vi "LV FPGA Serial Write.vi"(0 "Transmit":refnum<k21>="Port8/DIO0", 1 "Write FIFO":refnum<k21>="Write FIFO", 7 "baud rate (9600)":u32=9600, 9 "data bits (8)":i32=8 min=5 max=8 step=1, 11 "parity (0:none)":enum16{"None", "Odd", "Even", "Mark", "Space"}(ring), 12 "stop bits (10: 1 bit)":u16(ring)=10 items=["1.0"=10, "1.5"=15, "2.0"=20], 13 "Invert Polarity?":bool) -> ()   [LabVIEW 2009]
uses:
  <vilib>/eio/EIOMethodNode/EIOMethodNode.xnode
  <vilib>/rvi/eio/nirviEIOMethodImplementation/nirviEIOMethodImplementation.xnode
  <vilib>/rvi/eio/common/nirviEmuTemplateMethod_noerrors.vi
  <vilib>/rvi/eio/common/nirviEmuClasses.ctl
  <vilib>/rvi/DataTransferAndStorage/Container/XNode/niFpgaContainer.xnode
  <vilib>/rvi/DataTransferAndStorage/Container/Common/niFpgaContainerMethod.ctl
  <vilib>/rvi/DataTransferAndStorage/Container/Common/niFpgaContainerExecOnDevCompGetState.vi
  <vilib>/rvi/DataTransferAndStorage/Container/Common/niFpgaContainerMetaDataKey.ctl
  <vilib>/rvi/FIFO/Fifo_Resource/nirvififoUniquifyingName.vi
  <vilib>/rvi/interface/RandomDataEmulation/niFpgaRandomDataHandleErrors.vi
  <vilib>/rvi/interface/RandomDataEmulation/nirviRandomDataFPGAFIFO.vi
  <vilib>/rvi/DataTransferAndStorage/Container/Common/niFpgaTransferTypeControl.ctl
  <vilib>/rvi/DataTransferAndStorage/FIFO/niFpgaPeerToPeerStreamState.ctl
  <vilib>/rvi/eio/common/nirviEmuReportErrorAndStop.vi
  <vilib>/eio/EIONode/EIONode.xnode
  <vilib>/rvi/eio/nirviEIOImplementation/nirviEIOImplementation.xnode
panel:
  out "Read: Transmission Error":bool
  in  "stop":bool
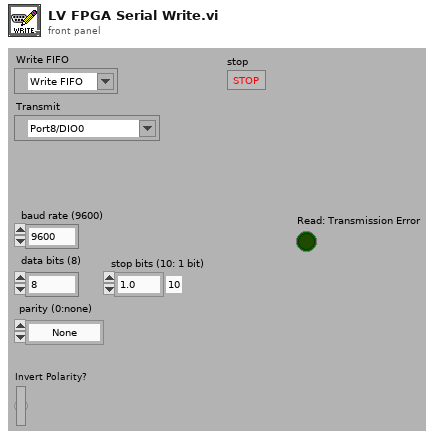
[diagram p1: front panel]
types:
  T1 = typedef "nirviEmuClasses.ctl" = enum16{"IO Read", "IO Write", "Method", "Property Read", "Property Write"}
  T2 = typedef "niFpgaContainerMethod.ctl" = enum16{"Write", "Read", "Clear", "Get Number of Elements to Write", "Get Number of Elements to Read", "Enable", "Disable", "Flush and Disable", "Get Stream State"}
  T3 = typedef "niFpgaTransferTypeControl.ctl" = enum16{"Target-Scoped", "Host to Target - DMA", "Target to Host - DMA", "Peer to Peer Reader", "Peer to Peer Writer", "Bidirectional"}
  T4 = typedef "niFpgaPeerToPeerStreamState.ctl" = enum16{"Unlinked", "Disabled", "Enabled", "Flushing"}
  T5 = typedef "niFpgaContainerMetaDataKey.ctl" = enum16{"FPGA FIFO", "FPGA Memory", "FPGA Register"}
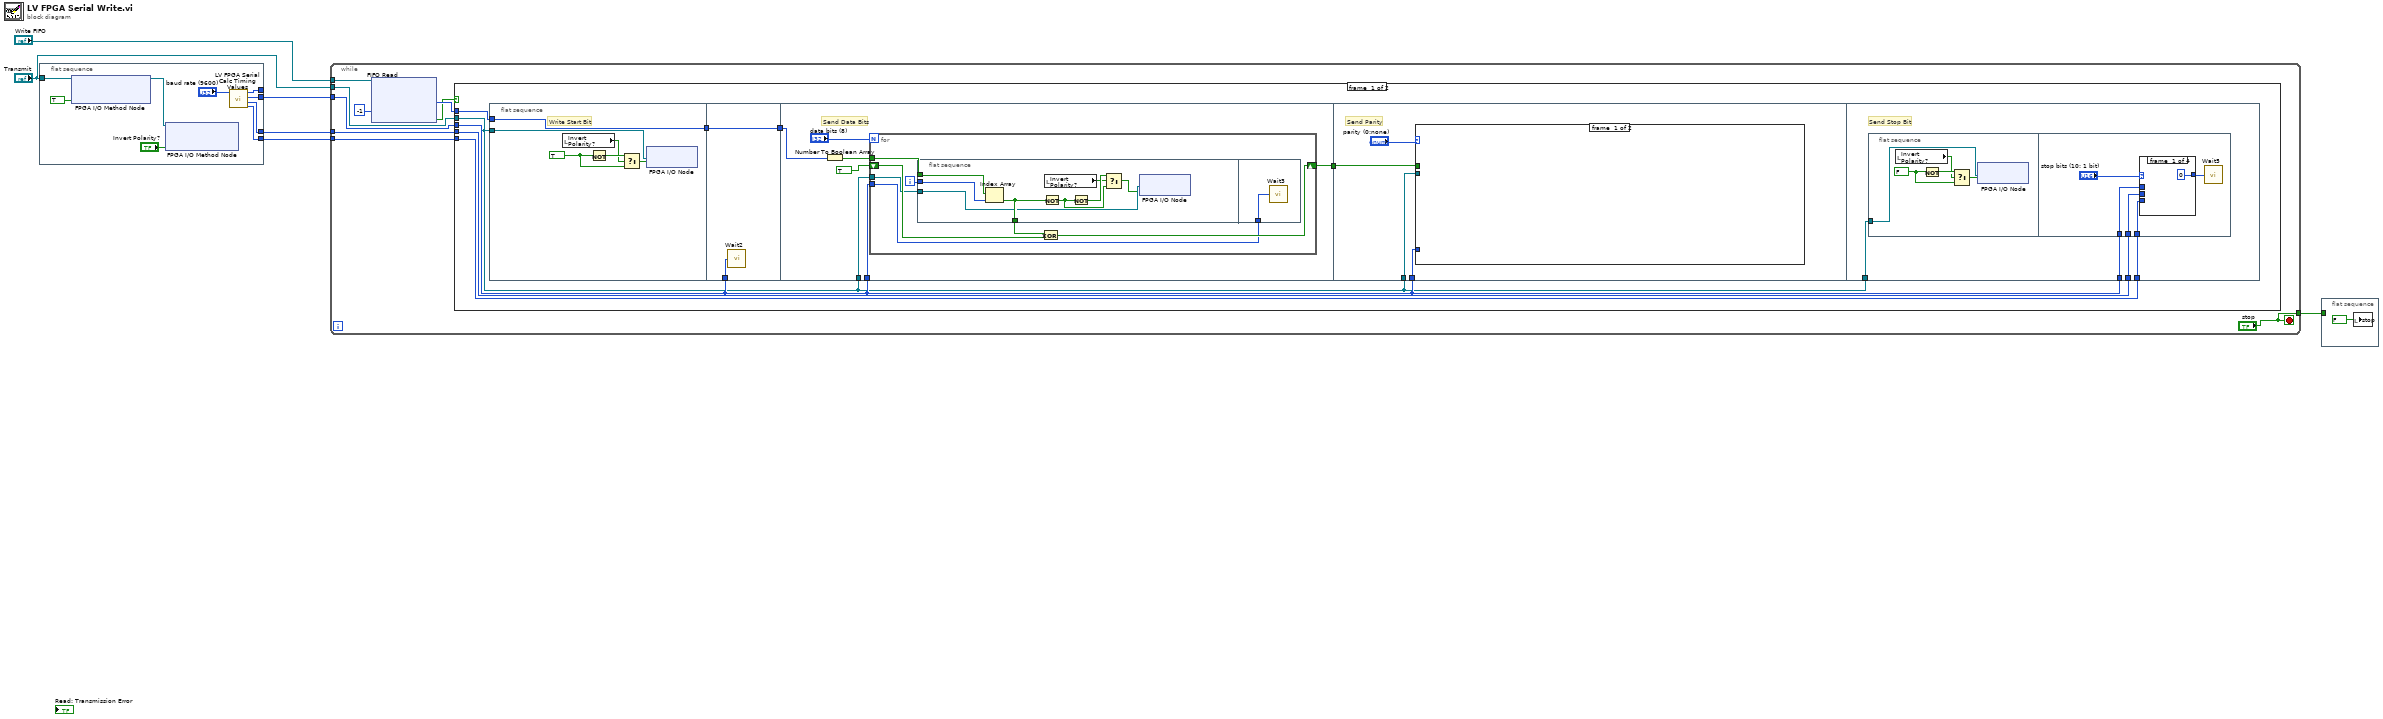
[diagram p0: block diagram]
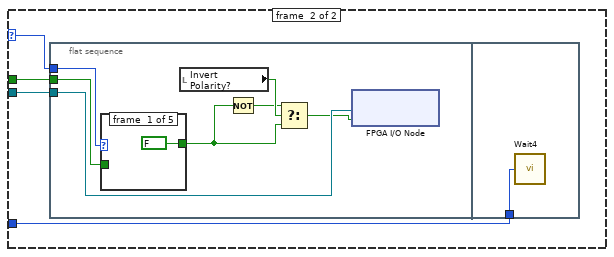
[diagram p2: hidden frame]
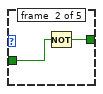
[diagram p3: hidden frame]
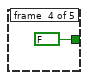
[diagram p5: hidden frame]
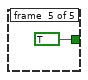
[diagram p6: hidden frame]
diagram:
  n1 = flat-sequence {
    tunnel: [w11] -> w6
    tunnel: [w14] -> _
    tunnel: [w13] -> w5
    tunnel: [w12] -> w4
    tunnel: "Transmit" -> [w9]
    frame #0 {
      n2 = xnode "FPGA I/O Method Node"("FPGA I/O In"=w9, "Enable"=TRUE ("Digital Enable")) -> ("FPGA I/O Out"=w8:refnum<k21>)
      n3 = xnode "FPGA I/O Method Node"("FPGA I/O In"=w8, "Data"="Invert Polarity?") -> ()  [unwired: 1 out]
      n4 = call "LV FPGA Serial Calc Timing Values.vi"("baud rate (1000000)"="baud rate (9600)") -> ("Two Bit"=w12:u32, "One and Half Bit"=w13:u32, "One Bit"=w11:u32, "Half Bit"=w14:u32)  [unwired: 1 in, 2 out]
    }
  }
  n5 = while {
    tunnel: w4 -> [w46]
    tunnel: w5 -> [w45]
    tunnel: w6 -> [w44]
    tunnel: "Transmit" -> [w43]
    tunnel: ["stop"] -> w2
    tunnel: "Write FIFO" -> [w39]
    stop <- "stop" stop-if-true
    n6 = xnode ("FIFO Read")("Timeout"=-1, "FIFO In"=w39) -> ("Element"=w42:u8, "Timed Out?"=w40:bool)  [unwired: 1 out]
    n7 = case shown="False" w40 {
      tunnel: w46 -> [w337 _]
      tunnel: w45 -> [w336 _]
      tunnel: w44 -> [w335 _]
      tunnel: w43 -> [w334 _]
      tunnel: w42 -> [w333 _]
      frame #0 {
        n8 = flat-sequence {
          tunnel: w334 -> [w346]
          tunnel: w333 -> [w341]
          tunnel: [w341] -> w340
          tunnel: w335 -> [w359]
          tunnel: [w358] -> w339
          tunnel: w340 -> [w358]
          tunnel: w335 -> [w366]
          tunnel: [w364] -> w338
          tunnel: w334 -> [w362]
          tunnel: w339 -> [w361]
          tunnel: w335 -> [w396]
          tunnel: w338 -> [w397]
          tunnel: w334 -> [w395]
          tunnel: w335 -> [w430]
          tunnel: w336 -> [w429]
          tunnel: w337 -> [w428]
          tunnel: w334 -> [w427]
          frame #0 {
            w344 = TRUE
            # "Write Start Bit"
            n9 = local read "Invert Polarity?"() -> (w343:bool)
            n10 = Not(x=w344) -> (.not. x?=w345:bool)
            n11 = Select(t=w345, s=w343, f=w344) -> (s? t:f=w342:bool)
            n12 = xnode "FPGA I/O Node"("I/O Item"=w342, "FPGA I/O In"=w346) -> ()  [unwired: 1 out]
          }
          frame #1 {
            n13 = call "Wait2"("Count(Ticks)"=w359) -> ()  [unwired: 1 out]
          }
          frame #2 {
            # "Send Data Bits"
            n14 = Number To Boolean Array(number=w361) -> (Boolean array=w363:bool[])
            n15 = for {
              N: "data bits (8)" -> [_]
              tunnel: w366 -> [w370]
              shift-right: [w373] -> w364
              shift-left: TRUE -> [w372]
              tunnel: w363 -> [w369]
              tunnel: w362 -> [w367]
              i -> [w371]
              n16 = flat-sequence {
                tunnel: w371 -> [w381]
                tunnel: w369 -> [w380]
                tunnel: [w379] -> w368
                tunnel: w367 -> [w378]
                tunnel: w370 -> [w393]
                frame #0 {
                  n17 = Index Array(array=w380, index=w381) -> (element=w379:bool)
                  n18 = Not(x=w379) -> (.not. x?=w376:bool)
                  n19 = local read "Invert Polarity?"() -> (w375:bool)
                  n20 = Not(x=w376) -> (.not. x?=w377:bool)
                  n21 = Select(t=w377, s=w375, f=w376) -> (s? t:f=w374:bool)
                  n22 = xnode "FPGA I/O Node"("I/O Item"=w374, "FPGA I/O In"=w378) -> ()  [unwired: 1 out]
                }
                frame #1 {
                  n23 = call "Wait3"("Count(Ticks)"=w393) -> ()  [unwired: 1 out]
                }
              }
              n24 = Exclusive Or(1:w372, 2:w368) -> (0:w373:bool)
            }
          }
          frame #3 {
            # "Send Parity"
            n25 = case shown="\"Odd\", Default" "parity (0:none)" {
              selector: "parity (0:none)" -> [_ w401]
              tunnel: w397 -> [_ w400]
              tunnel: w396 -> [_ w399]
              tunnel: w395 -> [_ w398]
              frame #0 {
              }
              frame #1 {
                n26 = flat-sequence {
                  tunnel: w400 -> [w407]
                  tunnel: w401 -> [w408]
                  tunnel: w398 -> [w406]
                  tunnel: w399 -> [w426]
                  frame #0 {
                    n27 = case shown="\"Even\"" w408 {
                      tunnel: w407 -> [_ w422 w423 _ _]
                      tunnel: [FALSE ("y") w421 w423 FALSE ("y") TRUE ("y")] -> w403
                      frame #0 {
                      }
                      frame #1 {
                        n28 = Not(x=w422) -> (.not. x?=w421:bool)
                      }
                      frame #2 {
                      }
                      frame #3 {
                      }
                      frame #4 {
                      }
                    }
                    n29 = local read "Invert Polarity?"() -> (w405:bool)
                    n30 = Not(x=w403) -> (.not. x?=w404:bool)
                    n31 = Select(t=w404, s=w405, f=w403) -> (s? t:f=w402:bool)
                    n32 = xnode "FPGA I/O Node"("I/O Item"=w402, "FPGA I/O In"=w406) -> ()  [unwired: 1 out]
                  }
                  frame #1 {
                    n33 = call "Wait4"("Count(Ticks)"=w426) -> ()  [unwired: 1 out]
                  }
                }
              }
            }
          }
          frame #4 {
            # "Send Stop Bit"
            n34 = flat-sequence {
              tunnel: w427 -> [w435]
              tunnel: w430 -> [w451]
              tunnel: w429 -> [w450]
              tunnel: w428 -> [w449]
              frame #0 {
                w433 = FALSE
                n35 = local read "Invert Polarity?"() -> (w432:bool)
                n36 = Not(x=w433) -> (.not. x?=w434:bool)
                n37 = Select(t=w434, s=w432, f=w433) -> (s? t:f=w431:bool)
                n38 = xnode "FPGA I/O Node"("I/O Item"=w431, "FPGA I/O In"=w435) -> ()  [unwired: 1 out]
              }
              frame #1 {
                n39 = case shown="20" "stop bits (10: 1 bit)" {
                  tunnel: w451 -> [_ w453 _ _]
                  tunnel: w450 -> [_ _ w454 _]
                  tunnel: w449 -> [_ _ _ w455]
                  tunnel: [u32 0 ("One Bit") w453 w454 w455] -> w448
                  frame #0 {
                  }
                  frame #1 {
                  }
                  frame #2 {
                  }
                  frame #3 {
                  }
                }
                n40 = call "Wait5"("Count(Ticks)"=w448) -> ()  [unwired: 1 out]
              }
            }
          }
        }
      }
      frame #1 {
      }
    }
  }
  n41 = flat-sequence {
    tunnel: w2 -> [_]
    frame #0 {
      n42 = local write "stop"(FALSE ("stop")) -> ()
    }
  }
